vi "Autotest.vi"(8 "error in (no error)":errorcluster caption="entrée d'erreur (pas d'erreur)", 11 "Class Relay_Board 16_Relay_CH340 en entrée":refnum<class "Class Relay_Board 16_Relay_Acer_Micro.lvclass">) -> (0 "error out":errorcluster caption="sortie d'erreur", 2 "Autotest Ok ?":bool, 3 "Class Relay_Board 16_Relay_CH340 en sortie":refnum<class "Class Relay_Board 16_Relay_Acer_Micro.lvclass">)   [LabVIEW 2020, in "Library Instrument & Equipement.lvlib" / "Library Relay_Board.lvlib" / "Class Relay_Board 16_Relay_Acer_Micro.lvclass"]
uses:
  Class Relay_Board 16_Relay_Acer_Micro.lvclass
  C:/Users/ngarcin/OneDrive - Altyor/Standard TB/Class/Relay_Board/Relay_Board (Default)/Class Relay_Board (Default).lvclass
  <vilib>/Instr/_visa.llb/VISA Find Search Mode.ctl
  Class Relay_Board 16_Relay_Acer_Micro.lvclass/Class Relay_Board 16_Relay_Acer_Micro.ctl
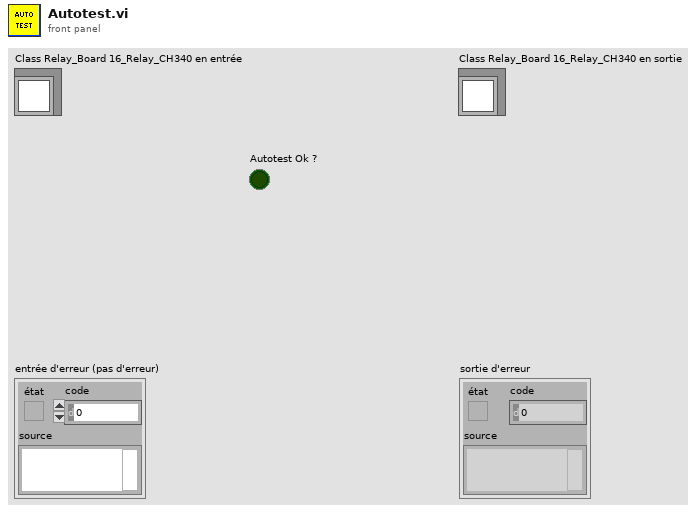
[diagram p1: front panel]
types:
  T1 = typedef "VISA Find Search Mode.ctl" = u32
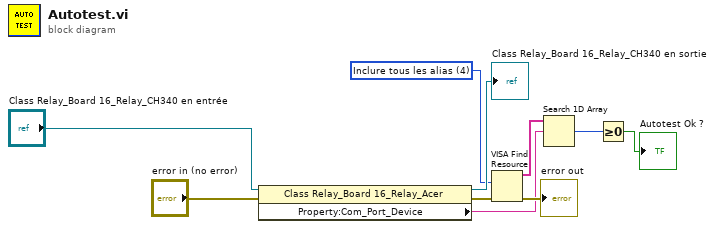
[diagram p0: block diagram]
diagram:
  w5 = T1 4 items=["Noms canoniques uniquement"=0, "Alias uniquement"=2, "Inclure les alias correspondants"=3, "Inclure tous les alias"=4] ("Search Mode")
  n1 = property class="Class Relay_Board 16_Relay_Acer"(reference="Class Relay_Board 16_Relay_CH340 en entrée", error in="error in (no error)") -> (reference out=→"Class Relay_Board 16_Relay_CH340 en sortie":refnum<class "Class Relay_Board 16_Relay_Acer_Micro.lvclass">, error out=w8:errorcluster, "Property:Com_Port_Device"=w4:string)
  n2 = VISA Find Resource(8:w8, 10:w5) -> (0:→"error out":errorcluster, 3:w3:string[])  [unwired: 1 in, 1 out]
  n3 = Search 1D Array(1D array=w3, element=w4) -> (index of element=w2:i32)  [unwired: 1 in]
  n4 = Greater Or Equal To 0?(x=w2) -> (x >= 0?=→"Autotest Ok ?":bool)
